vi "ConfigureLights (SubVI).vi"(7 "Power Supply GPIB Address":string="8") -> ()   [LabVIEW 2016]
doc: "Send commands with the GPIB Write function. Read the response from the instrument with the GPIB Read function.\n\nThis VI configures the power supply at the channel level to set up the lighting for the image samples. It sends voltage and current related commands.\n\nThe power supply is compatible with IEEE-488/2 and SCPI standards according to the manufacturer. Commands take the form of writes or queries. Semicolon, ';', concatenates commands.\n\nOverview: Configures the programmable power supply for the lightson the camera mount. Built from the \"Simple GPIB\" NI example. (Demonstrates the use of the GPIB functions to communicate to a GPIB instrument.)\n\nRequirements: NI-488.2 Driver\nInstructions:\nEnsure the programmable power supply (GW Instek's PST-3202) is connected with the specified GPIB Address matching the control. Configure properly through Measurement & Automation Explorer.\n\nIn this VI, we assume that the primary light source is connected to the power supply via Channel 1, while the secondary light source, the spotlight, is connected on Channel 2. Our commands translate as follows: \n\nCHAN1:PROT:VOLT 7.1; PROT:VOLT? -- Set the overvoltage protection on channel 1 to 7.1 V, then check the overvoltage protection setting.\n\nCHAN1:CURR 0.015; CURR? -- Set the current to 15mA on channel 1, then check the current setting. \n\nCHAN1:PROT:CURR 0; PROT:CURR? -- turn on the overcurrent protection in channel 1, then check the overcurrent protection setting.\n\nAnother VI, _______, serves as the slow control for monitoring the output voltage. An additional VI, LightSwitch, simply switches the lights on and off by manipulating the voltage on each channel."
panel:
  out "Response":string
  # "Overview: Configures the programmable power supply  for the lightson the camera mount.  Built from the \"Simple GPIB\" NI example. (Demonstrates the use of the GPIB functions to communicate to a GPIB instrument.)\n\nRequirements: NI-488.2 Driver\nInstructions:\nEnsure the programmable power supply (GW Instek's PST-3202) is connected with the specified GPIB Address matching the control. Configure properly through Measurement & Automation Explorer."
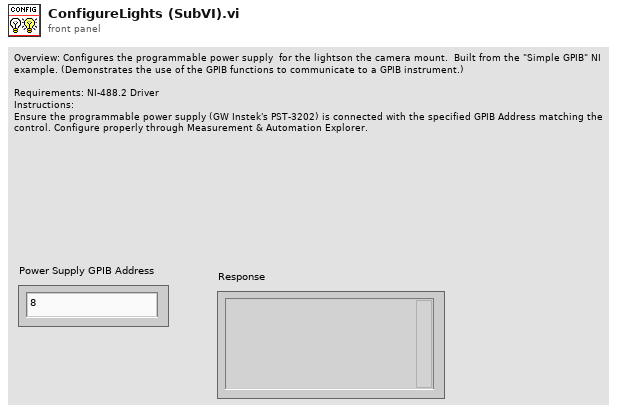
[diagram p1: front panel]
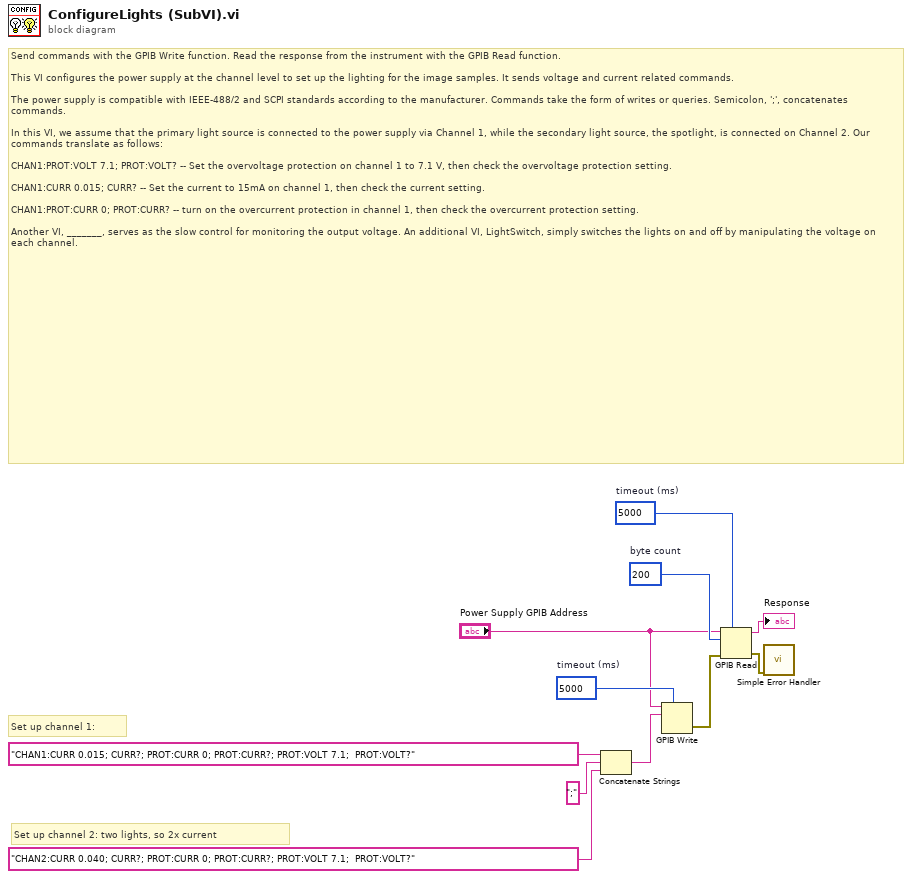
[diagram p0: block diagram]
diagram:
  w5 = 5000  # timeout (ms)
  w8 = 200  # byte count
  w7 = 5000  # timeout (ms)
  # "Set up channel 2: two lights, so 2x current"
  # "Set up channel 1:"
  # "Send commands with the GPIB Write function. Read the response from the instrument with the GPIB Read function.\n\nThis VI configures the power supply at the channel level to set up the lighting for the image samples. It sends voltage and current related commands.\n\nThe power supply is compatible with IEEE-488/2 and SCPI standards according to the manufacturer. Commands take the form of writes or queries. Semicolon, ';', concatenates commands.\n\nIn this VI, we assume that the primary light source is connected to the power supply via Channel 1, while the secondary light source, the spotlight, is connected on Channel 2. Our commands translate as follows: \n\nCHAN1:PROT:VOLT 7.1; PROT:VOLT? -- Set the overvoltage protection on channel 1 to 7.1 V, then check the overvoltage protection setting.\n\nCHAN1:CURR 0.015; CURR? -- Set the current to 15mA on channel 1, then check the current setting. \n\nCHAN1:PROT:CURR 0; PROT:CURR? -- turn on the overcurrent protection in channel 1, then check the overcurrent protection setting.\n\nAnother VI, _______, serves as the slow control for monitoring the output voltage. An additional VI, LightSwitch, simply switches the lights on and off by manipulating the voltage on each channel."
  n1 = Concatenate Strings("CHAN1:CURR 0.015; CURR?; PROT:CURR 0; PROT:CURR?; PROT:VOLT 7.1;  PROT:VOLT?" ("Characters to Write"), ";" ("string"), "CHAN2:CURR 0.040; CURR?; PROT:CURR 0; PROT:CURR?; PROT:VOLT 7.1;  PROT:VOLT?" ("Characters to Write")) -> (w3:string)
  n2 = GPIB Write(0:"Power Supply GPIB Address", 1:w3, 4:w7) -> (6:w10:errorcluster)  [unwired: 2 in, 1 out]
  n3 = GPIB Read(0:"Power Supply GPIB Address", 1:w8, 3:w10, 4:w5) -> (5:→"Response":string, 7:w9:errorcluster)  [unwired: 1 in, 1 out]
  n4 = call <vilib>:"Simple Error Handler.vi"("error in (no error)"=w9) -> ()  [unwired: 4 in, 5 out]
